vi "WFS Zernike Lsf.vi"(8 "error in (no error)":errorcluster {"code" format="%.0x"}, 10 "Zernike Orders":i32, 11 "instrument handle":refnum<visa-resource-name>) -> (0 "error out":errorcluster {"code" format="%.0x"}, 1 "Array Zernike um":sgl[](array[numeric]) format="%.2p", 3 "instrument handle out":refnum<visa-resource-name>, 4 "Array Zernike Orders um":sgl[](array[numeric]) format="%.2p", 5 "RoC mm":dbl)   [LabVIEW 2020]
doc: "This VI calculates the spot deviations (centroid with respect to its reference) and performs a least square fit to the desired number of Zernike VIs.\n\nOutput results are the Zernike coefficients up to the desired number of Zernike modes and an array summarizing these coefficients to rms amplitudes for each Zernike order."
uses:
  WFS_32.dll
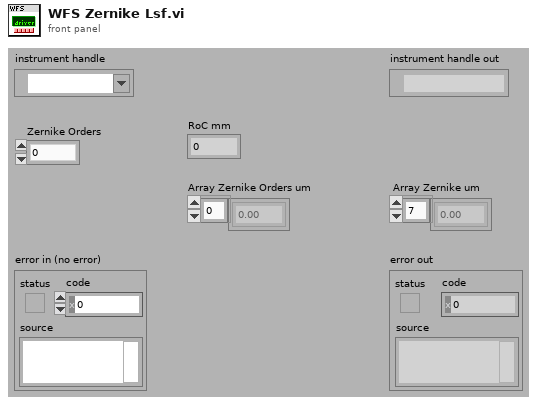
[diagram p1: front panel]
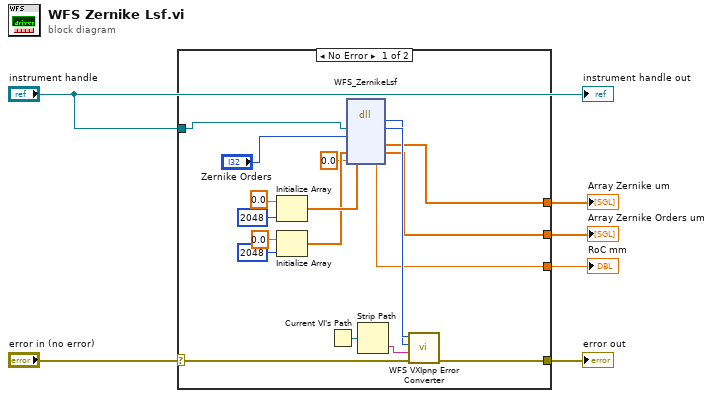
[diagram p0: block diagram]
diagram:
  n1 = case shown="No Error" "error in (no error)" {
    selector: "error in (no error)" -> [w19 w25]
    tunnel: [w18 w25] -> w6
    tunnel: "instrument handle" -> [w23 _]
    tunnel: [w14 _] -> w3
    tunnel: [w10 _] -> w2
    tunnel: [w8 _] -> w1
    frame No Error {
      n2 = Initialize Array(sgl 0.0 ("element"), 2048 ("dimension size")) -> (w17:sgl[])
      n3 = Initialize Array(sgl 0.0 ("element"), 2048 ("dimension size")) -> (w13:sgl[])
      n4 = Current VI's Path() -> (path=w24:path)
      n5 = dll-call lib="WFS_*.*" fn="WFS_ZernikeLsf"("Instrument Handle"=w23, "Zernike Orders"="Zernike Orders", "Array Zernike um"=w17, "Array Zernike Orders um"=w13, "RoC mm"=0.0) -> (w21:i32, "Instrument Handle"=w22:u32, "Array Zernike um"=w14:sgl[], "Array Zernike Orders um"=w10:sgl[], "RoC mm"=w8:dbl)  [unwired: 4 in, 2 out]
      n6 = Strip Path(path=w24) -> (name=w20:string)  [unwired: 1 out]
      n7 = call "WFS VXIpnp Error Converter.vi"("error in (no error)"=w19, "Name Of VI (\"\")"=w20, "CVI Error Code (0)"=w21, "instrument handle"=w22) -> ("error out"=w18:errorcluster)  [unwired: 6 in, 1 out]
    }
    frame Error {
    }
  }
  "error out" <- w6
  "Array Zernike um" <- w3
  "Array Zernike Orders um" <- w2
  "RoC mm" <- w1
  "instrument handle out" <- "instrument handle"
